vi "tap_stimulus_generator.vi"(1 "input cluster":T1) -> (0 "output cluster":T2)   [LabVIEW 2010]
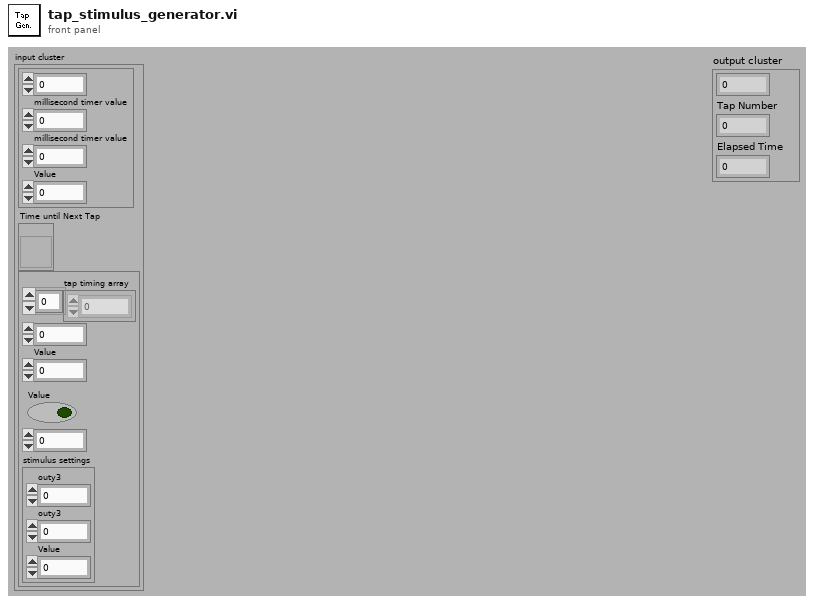
[diagram p1: front panel]
types:
  T1 = cluster{cluster{u32, "millisecond timer value":u32, "millisecond timer value":u32, "Value":u32}, "Time until Next Tap":refnum<vi>, cluster{"tap timing array":dbl[], i32, "Value":i32, "Value":bool, i32, "stimulus settings":cluster{"outy3":sgl, "outy3":i32, "Value":i32}}}
  T2 = cluster{i32, "Tap Number":i32, "Elapsed Time":i32}
  T3 = cluster{u32, "millisecond timer value":u32, "millisecond timer value":u32, "Value":u32}
  T4 = cluster{"tap timing array":dbl[], i32, "Value":i32, "Value":bool, i32, "stimulus settings":cluster{"outy3":sgl, "outy3":i32, "Value":i32}}
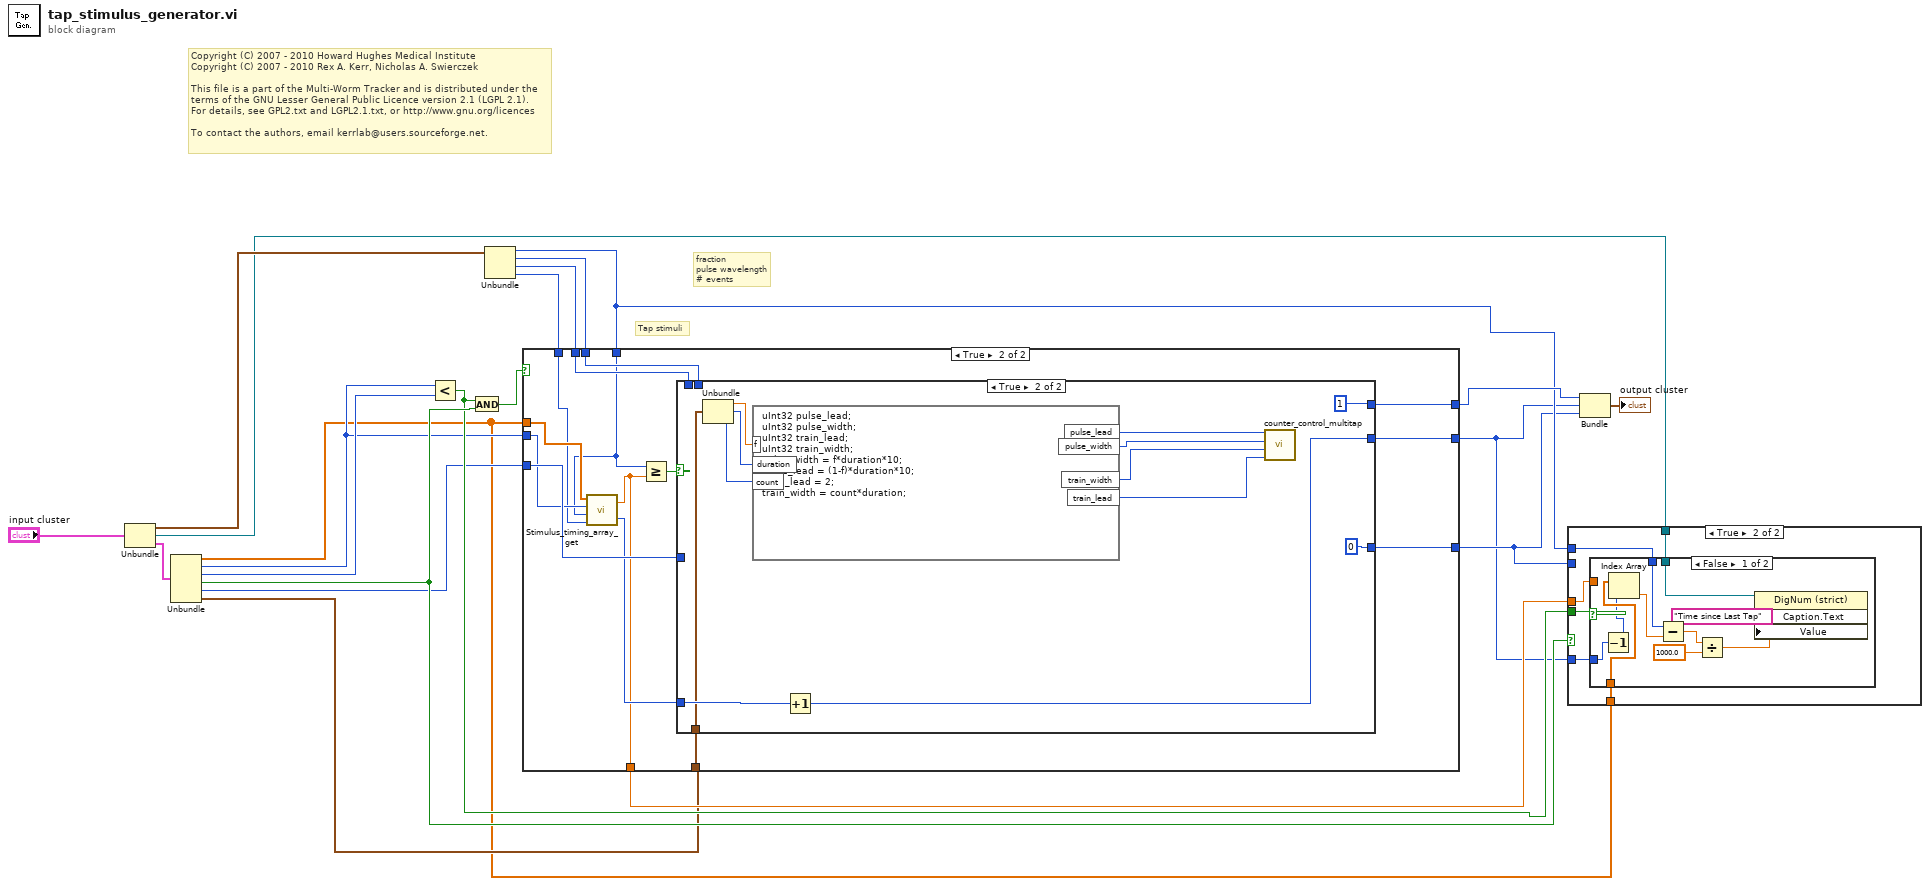
[diagram p0: block diagram]
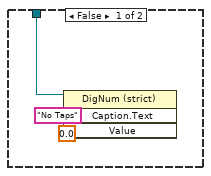
[diagram p2: hidden frame]
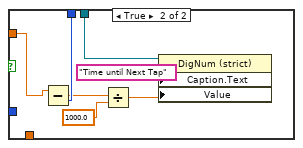
[diagram p3: hidden frame]
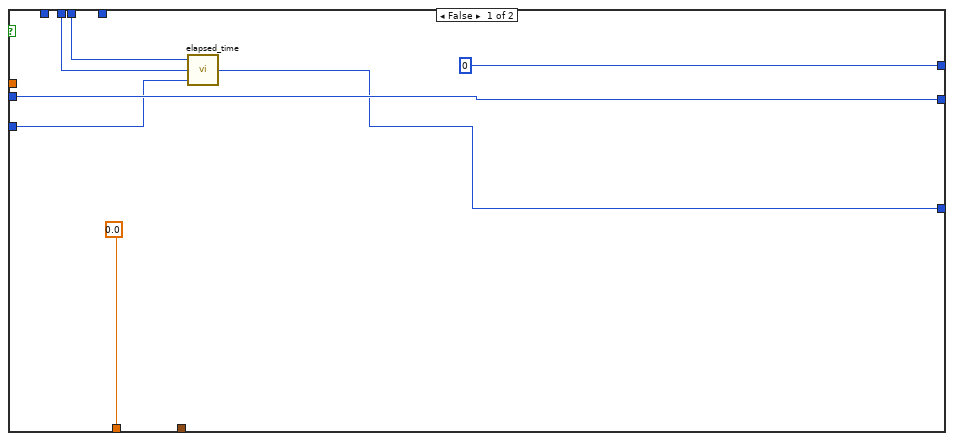
[diagram p4: hidden frame]
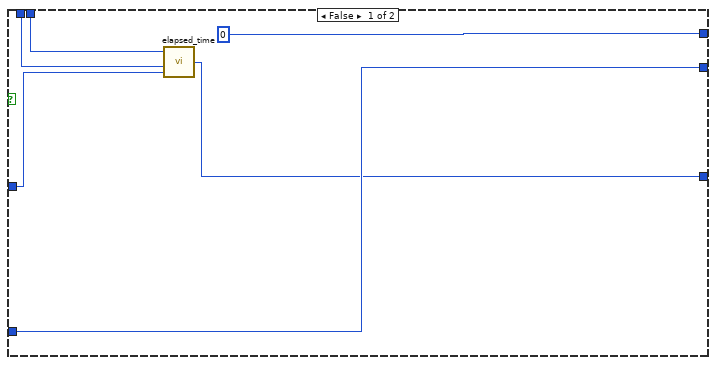
[diagram p5: hidden frame]
diagram:
  # "Copyright (C) 2007 - 2010 Howard Hughes Medical Institute\nCopyright (C) 2007 - 2010 Rex A. Kerr, Nicholas A. Swierczek\n \nThis file is a part of the Multi-Worm Tracker and is distributed under the\nterms of the GNU Lesser General Public Licence version 2.1 (LGPL 2.1).\nFor details, see GPL2.txt and LGPL2.1.txt, or http://www.gnu.org/licences\n \nTo contact the authors, email kerrlab@users.sourceforge.net."
  # "fraction\npulse wavelength\n# events"
  # "Tap stimuli"
  n1 = Unbundle("input cluster") -> (w19:T3, "Time until Next Tap"=w18:refnum<vi>, w17:T4)
  n2 = Unbundle(w17) -> ("tap timing array"=w2:dbl[], w9:i32, "Value"=w12:i32, "Value"=w16:bool, w14:i32, "stimulus settings"=w11:cluster{"outy3":sgl, "outy3":i32, "Value":i32})
  n3 = Less?(x=w9, y=w12) -> (x < y?=w15:bool)
  n4 = And(x=w15, y=w16) -> (x .and. y?=w21:bool)
  n5 = Unbundle(w19) -> (w6:u32, "millisecond timer value"=w7:u32, "millisecond timer value"=w8:u32, "Value"=w3:u32)
  n6 = case shown="True" w21 {
    tunnel: w2 -> [_ w33]
    tunnel: w9 -> [w28 w32]
    tunnel: [w28 w40] -> w1
    tunnel: w14 -> [w24 w35]
    tunnel: [w23 w41] -> w5
    tunnel: w7 -> [w26 w39]
    tunnel: w8 -> [w25 w38]
    tunnel: [0 w37] -> w13
    tunnel: [0.0 ("element") w30] -> w20
    tunnel: w11 -> [_ w36]
    tunnel: w6 -> [_ w31]
    tunnel: w3 -> [_ w29]
    frame False {
      n7 = call "elapsed_time.vi"("Time since last update"=w24, "Initial Time"=w25, "Current Time"=w26) -> ("Elapsed Time"=w23:i32)
    }
    frame True {
      n8 = call "Stimulus_timing_array_get.vi"("minimum time between events"=w29, "experiment time"=w31, "array index"=w32, "timing array"=w33) -> ("index"=w34:i32, "time"=w30:dbl)
      n9 = Greater Or Equal?(x=w31, y=w30) -> (x >= y?=w42:bool)
      n10 = case shown="True" w42 {
        tunnel: [w46 0] -> w41
        tunnel: w34 -> [w48 w59]
        tunnel: [w48 w58] -> w40
        tunnel: w35 -> [w45 _]
        tunnel: w39 -> [w43 _]
        tunnel: w38 -> [w44 _]
        tunnel: [0 1] -> w37
        tunnel: w36 -> [_ w56]
        frame False {
          n11 = call "elapsed_time.vi"("Time since last update"=w45, "Initial Time"=w44, "Current Time"=w43) -> ("Elapsed Time"=w46:i32)
        }
        frame True {
          n12 = Unbundle(w56) -> ("outy3"=w55:sgl, "outy3"=w54:i32, "Value"=w53:i32)
          n13 = formula code="uInt32 pulse_lead;\nuInt32 pulse_width;\nuInt32 train_lead;\nuInt32 train_width;\npulse_width = f*duration*10;\npulse_lead = (1-f)*duration*10;\ntrain_lead = 2;\ntrain_width = count*duration;"("f"=w55, "duration"=w54, "count"=w53) -> ("pulse_lead"=w52:u32, "pulse_width"=w51:u32, "train_lead"=w49:u32, "train_width"=w50:u32)
          n14 = Increment(x=w59) -> (x+1=w58:i32)
          n15 = call "counter_control_multitap.vi"("Downtime for pulse active"=w49, "Duration Pulse active"=w50, "Signal-high duration"=w51, "Signal-high lead-up"=w52) -> ()
        }
      }
    }
  }
  n16 = case shown="True" w16 {
    tunnel: w15 -> [_ w69]
    tunnel: w20 -> [_ w68]
    tunnel: w6 -> [_ w66]
    tunnel: w18 -> [w61 w67]
    tunnel: w5 -> [_ _]
    tunnel: w2 -> [_ w65]
    tunnel: w1 -> [_ w64]
    frame False {
      n17 = property on="Property Node" class="DigNum (strict)"(reference=w61, "Caption.Text"="No Taps" ("Label.Text"), "Value"=0.0 ("Time until Next Tap")) -> ()  [unwired: 1 in, 2 out]
    }
    frame True {
      n18 = case shown="False" w69 {
        tunnel: w68 -> [_ w84]
        tunnel: w66 -> [w70 w85]
        tunnel: w67 -> [w76 w80]
        tunnel: w65 -> [w73 _]
        tunnel: w64 -> [w74 _]
        frame False {
          n19 = Decrement(x=w74) -> (x-1=w72:i32)
          n20 = Index Array(array=w73, index=w72) -> (element=w71:dbl)
          n21 = Subtract(x=w70, y=w71) -> (x-y=w75:dbl)
          n22 = Divide(x=w75, y=1000.0) -> (x/y=w77:dbl)
          n23 = property on="Property Node" class="DigNum (strict)"(reference=w76, "Caption.Text"="Time since Last Tap" ("Label.Text"), "Value"=w77) -> ()  [unwired: 1 in, 2 out]
        }
        frame True {
          n24 = Subtract(x=w84, y=w85) -> (x-y=w83:dbl)
          n25 = Divide(x=w83, y=1000.0) -> (x/y=w81:dbl)
          n26 = property on="Property Node" class="DigNum (strict)"(reference=w80, "Caption.Text"="Time until Next Tap" ("Label.Text"), "Value"=w81) -> ()  [unwired: 1 in, 2 out]
        }
      }
    }
  }
  n27 = Bundle(w13, "index"=w1, "Elapsed Time"=w5) -> (→"output cluster":cluster{i32, "index":i32, "Elapsed Time":i32})  [unwired: 1 in]
